vi "practica_29_ grafica.vi"() -> ()   [LabVIEW 2019]
panel:
  out "XY Graph":cluster{dbl[], dbl[]}(graph)
  out "Eje Y":dbl[](array[numeric])
  out "Eje X":dbl[](array[numeric])
  out "Incremento":dbl
  in  "Nº Intervalos":i32
  out "XN":dbl
  out "X0":dbl
  # "Gráfica para la ecuación Y=5(1-e^-t/2)"
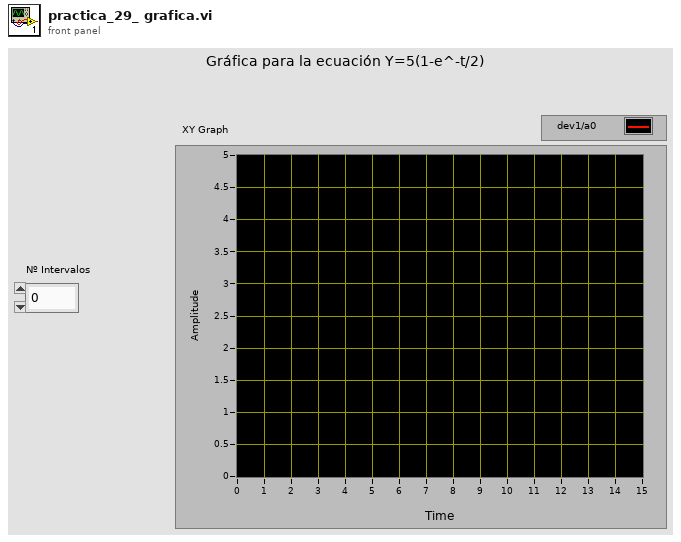
[diagram p1: front panel]
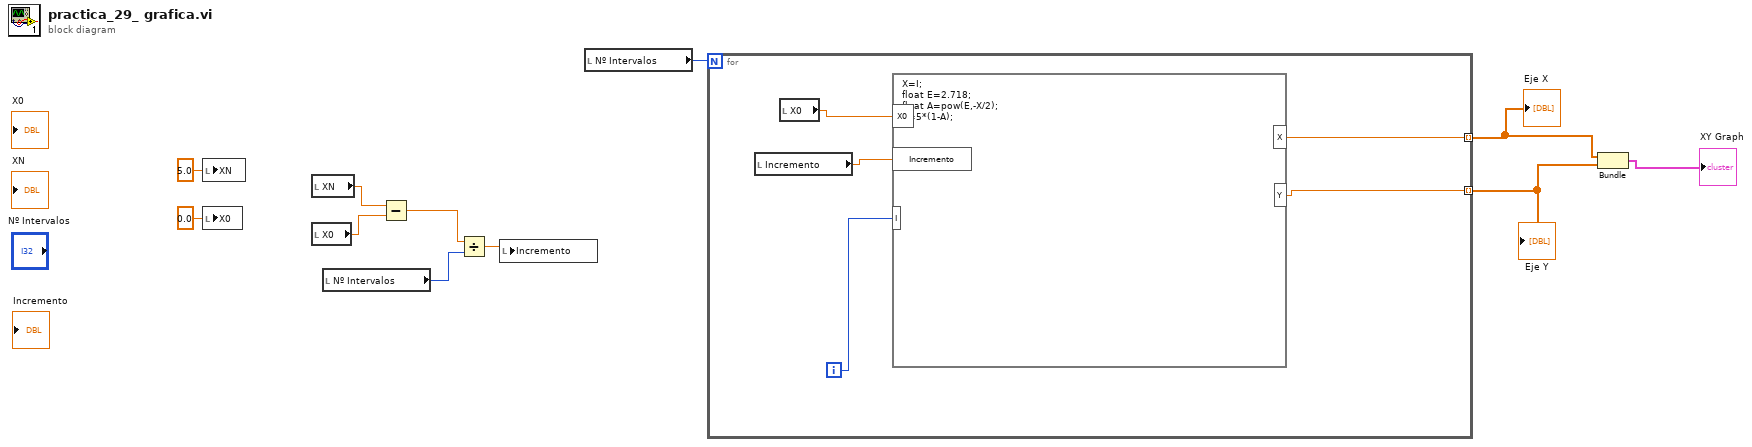
[diagram p0: block diagram]
diagram:
  n1 = local write "XN"(5.0 ("XN")) -> ()
  n2 = local write "X0"(0.0 ("X0")) -> ()
  n3 = local read "XN"() -> (w9:dbl)
  n4 = local read "X0"() -> (w8:dbl)
  n5 = local read "Nº Intervalos"() -> (w6:i32)
  n6 = Subtract(x=w9, y=w8) -> (x-y=w7:dbl)
  n7 = Divide(x=w7, y=w6) -> (x/y=w5:dbl)
  n8 = local write "Incremento"(w5) -> ()
  n9 = local read "Nº Intervalos"() -> (w4:i32)
  n10 = for {
    N: w4 -> [_]
    tunnel: [w13] -> w3 mode=indexing
    tunnel: [w12] -> w2 mode=indexing
    i -> [w16]
    n11 = local read "Incremento"() -> (w15:dbl)
    n12 = local read "X0"() -> (w14:dbl)
    n13 = formula code="X=I;\nfloat E=2.718;\nfloat A=pow(E,-X/2);\nY=5*(1-A);"("X0"=w14, "Incremento"=w15, "I"=w16) -> ("X"=w13:dbl, "Y"=w12:dbl)
  }
  "Eje X" <- w3
  "Eje Y" <- w2
  n14 = Bundle(w3, w2) -> (→"XY Graph":cluster{dbl[], dbl[]})  [unwired: 1 in]
